vi "LV FPGA Serial Read Write v1_1.vi"(5 "Receive":refnum<k21>="ConnectorA/DIO10", 7 "baud rate (9600)":u32=31250, 9 "data bits (8)":i32=8 min=5 max=8 step=1, 11 "parity (0:none)":enum16{"None", "Odd", "Even", "Mark", "Space"}(ring), 12 "stop bits (10: 1 bit)":u16(ring)=10 items=["1.0"=10, "1.5"=15, "2.0"=20], 13 "Invert Polarity?":bool) -> ()   [LabVIEW 2014]
uses:
  <vilib>/rvi/Emulation/niFpgaGetClockAttributes.vi
  <vilib>/rvi/Emulation/niFpgaSctlEmulationGetInTimedLoop.vi
  <vilib>/rvi/Emulation/niFpgaEmulationReportErrorSimple.vi
  <vilib>/rvi/Emulation/niFpgaProcessEmulError.vi
  Controls/Stop.vi
  <vilib>/rvi/eio/common/nirviEmuTemplateMethod_errors.vi
  <vilib>/rvi/Emulation/niFpgaCriticalErrorInLSC.vi
  <vilib>/rvi/Emulation/niFpgaEmulationIsFPGAContextNoSignature.vi
  <vilib>/rvi/errors/niFpgaSetErrorForExecOnDevCompSimple.vi
  <vilib>/rvi/eio/common/nirviEmuReportErrorAndStop.vi
  <vilib>/rvi/DataTransferAndStorage/Container/Common/niFpgaContainerGetUniqueNameForEmu.vi
  <vilib>/rvi/FIFO/Fifo_Resource/nirvififoEmulationSetSize.vi
  <vilib>/rvi/FIFO/Fifo_Resource/nirviFifoEmulationQueueMgr.vi
  <instcachedir>/0/nirviFifoEmulationQueueMgr_E5CAEC123FF24DC58D834DCA3CDAA9B5.lvgen/nirviFifoEmulationQueueMgr_E5CAEC123FF24DC58D834DCA3CDAA9B5_000.vi
  <vilib>/rvi/FIFO/Fifo_Resource/nirvififoEmulationDetermineInputValidOut.vi
  <vilib>/rvi/FIFO/Fifo_Resource/nirvififoEmulationCreateLock.vi
  <vilib>/rvi/FIFO/Fifo_Resource/nirvififoEmulationObtainLock.vi
  <vilib>/rvi/FIFO/Fifo_Resource/nirvififoEmulationReleaseLock.vi
  <vilib>/rvi/occurrence/nirviWaitOnOccurrenceBase.vi
  <vilib>/rvi/errors/nirviReportUnexpectedCaseInternalError.vi
  <vilib>/rvi/errors/nirviReportUnexpectedCaseInternalError (U32).vi
  <vilib>/eio/EIONode/EIONode.xnode
  <vilib>/rvi/DataTransferAndStorage/Container/XNode/niFpgaContainer.xnode
  <vilib>/rvi/FIFO/Fifo_Resource/nirvififoEmulationWrite.vi
panel:
  out "Read: Transmission Error":bool
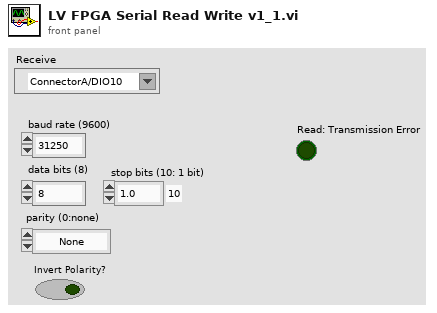
[diagram p1: front panel]
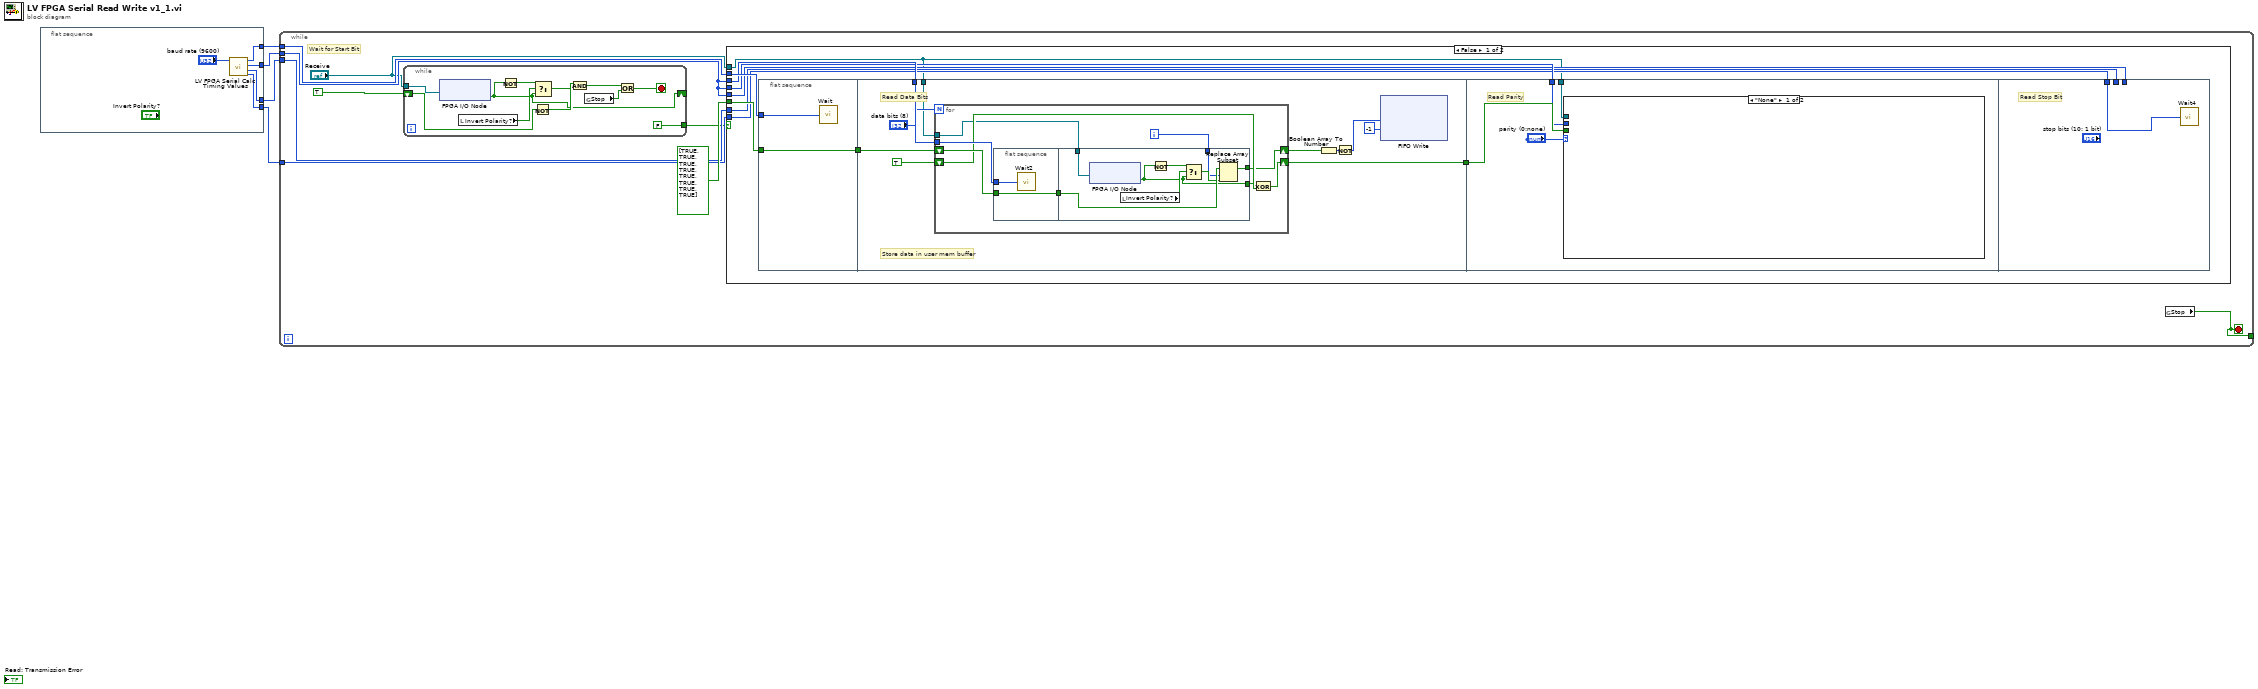
[diagram p0: block diagram]
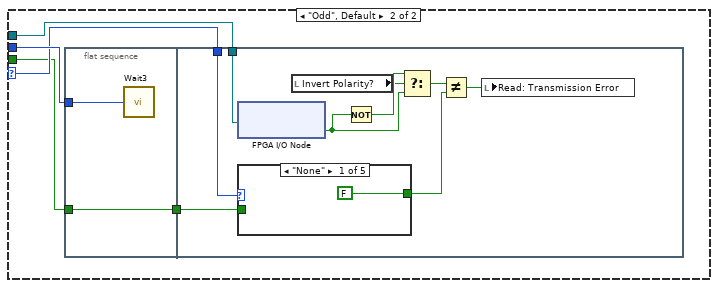
[diagram p2: hidden frame]
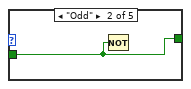
[diagram p3: hidden frame]
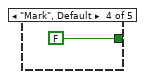
[diagram p5: hidden frame]
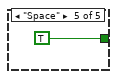
[diagram p6: hidden frame]
diagram:
  n1 = flat-sequence {
    tunnel: [w5] -> w3
    tunnel: [w8] -> w4
    tunnel: [w7] -> w2
    tunnel: [w6] -> w1
    frame #0 {
      n2 = call "LV FPGA Serial Calc Timing Values.vi"("baud rate (1000000)"="baud rate (9600)") -> ("Two Bit"=w6:u32, "One and Half Bit"=w7:u32, "One Bit"=w5:u32, "Half Bit"=w8:u32)  [unwired: 1 in, 2 out]
    }
  }
  n3 = while {
    tunnel: w1 -> [w17]
    tunnel: w2 -> [w16]
    tunnel: w3 -> [w15]
    tunnel: w4 -> [w14]
    tunnel: [w10] -> _
    stop <- w10 stop-if-true
    # "Wait for Start Bit"
    n4 = while {
      tunnel: [FALSE] -> w13
      shift-right: [w20] -> _
      shift-left: TRUE -> [w28]
      tunnel: "Receive" -> [w24]
      stop <- w25 stop-if-true
      n5 = xnode "FPGA I/O Node"("FPGA I/O In"=w24) -> ("I/O Item"=w20:bool)  [unwired: 1 out]
      n6 = local read "Invert Polarity?"() -> (w22:bool)
      n7 = Not(x=w20) -> (.not. x?=w23:bool)
      n8 = Not(x=w28) -> (.not. x?=w27:bool)
      n9 = Select(t=w23, s=w22, f=w20) -> (s? t:f=w21:bool)
      n10 = And(x=w27, y=w21) -> (x .and. y?=w26:bool)
      n11 = global read "Stop.vi" "Stop"() -> (w19:bool)
      n12 = Or(x=w26, y=w19) -> (x .or. y?=w25:bool)
    }
    n13 = case shown="False" w13 {
      tunnel: bool[] [TRUE, TRUE, TRUE, TRUE, TRUE, TRUE, TRUE, TRUE] -> [w38 _]
      tunnel: w14 -> [w37 _]
      tunnel: w15 -> [w36 _]
      tunnel: w15 -> [w35 _]
      tunnel: w15 -> [w34 _]
      tunnel: w16 -> [w33 _]
      tunnel: w17 -> [w32 _]
      tunnel: "Receive" -> [w30 _]
      frame False {
        n14 = flat-sequence {
          tunnel: [w41] -> w39
          tunnel: w38 -> [w41]
          tunnel: w37 -> [w40]
          tunnel: w39 -> [w51]
          tunnel: w36 -> [w50]
          tunnel: [w48] -> w31
          tunnel: w30 -> [w46]
          tunnel: w35 -> [w72]
          tunnel: w31 -> [w74]
          tunnel: w30 -> [w71]
          tunnel: w34 -> [_]
          tunnel: w33 -> [_]
          tunnel: w32 -> [w96]
          frame #0 {
            n15 = call "Wait"("Count(Ticks)"=w40) -> ()  [unwired: 1 out]
          }
          frame #1 {
            # "Store data in user mem buffer"
            # "Read Data Bits"
            n16 = for {
              N: "data bits (8)" -> [_]
              shift-right: [w54] -> w42
              shift-left: w51 -> [w60]
              tunnel: w50 -> [w58]
              shift-right: [w57] -> w48
              shift-left: TRUE -> [w56]
              tunnel: w46 -> [w53]
              i -> [w52]
              n17 = flat-sequence {
                tunnel: w60 -> [w62]
                tunnel: [w62] -> w59
                tunnel: w58 -> [w61]
                tunnel: w59 -> [w70]
                tunnel: [w69] -> w54
                tunnel: [w64] -> w55
                tunnel: w53 -> [w68]
                tunnel: w52 -> [w63]
                frame #0 {
                  n18 = call "Wait2"("Count(Ticks)"=w61) -> ()  [unwired: 1 out]
                }
                frame #1 {
                  n19 = xnode "FPGA I/O Node"("FPGA I/O In"=w68) -> ("I/O Item"=w64:bool)  [unwired: 1 out]
                  n20 = local read "Invert Polarity?"() -> (w67:bool)
                  n21 = Not(x=w64) -> (.not. x?=w66:bool)
                  n22 = Select(t=w66, s=w67, f=w64) -> (s? t:f=w65:bool)
                  n23 = Replace Array Subset(array=w70, new element=w65, index=w63) -> (w69:bool[])
                }
              }
              n24 = Exclusive Or(1:w56, 2:w55) -> (0:w57:bool)
            }
            n25 = Boolean Array To Number(Boolean array=w42) -> (number=w44:u8)
            n26 = Not(x=w44) -> (.not. x?=w43:u8)
            n27 = xnode ("FIFO Write")("Element"=w43, "Timeout"=-1) -> ()  [unwired: 1 in, 2 out]
          }
          frame #2 {
            # "Read Parity"
            n28 = case shown="\"None\"" "parity (0:none)" {
              selector: "parity (0:none)" -> [_ w78]
              tunnel: w74 -> [_ w76]
              tunnel: w72 -> [_ w79]
              tunnel: w71 -> [_ w75]
              frame "None" {
              }
              frame "Odd", Default {
                n29 = flat-sequence {
                  tunnel: w79 -> [w81]
                  tunnel: [w80] -> w77
                  tunnel: w76 -> [w80]
                  tunnel: w78 -> [w90]
                  tunnel: w77 -> [w88]
                  tunnel: w75 -> [w86]
                  frame #0 {
                    n30 = call "Wait3"("Count(Ticks)"=w81) -> ()  [unwired: 1 out]
                  }
                  frame #1 {
                    n31 = xnode "FPGA I/O Node"("FPGA I/O In"=w86) -> ("I/O Item"=w83:bool)  [unwired: 1 out]
                    n32 = case shown="\"None\"" w90 {
                      tunnel: w88 -> [_ w92 w93 _ _]
                      tunnel: [FALSE ("y") w92 w93 FALSE ("y") TRUE ("y")] -> w89
                      frame "None" {
                      }
                      frame "Odd" {
                        n33 = Not(x=w92) -> ()  [unwired: 1 out]
                      }
                      frame "Even" {
                      }
                      frame "Mark", Default {
                      }
                      frame "Space" {
                      }
                    }
                    n34 = local read "Invert Polarity?"() -> (w84:bool)
                    n35 = Not(x=w83) -> (.not. x?=w85:bool)
                    n36 = Select(t=w85, s=w84, f=w83) -> (s? t:f=w82:bool)
                    n37 = Not Equal?(x=w82, y=w89) -> (x != y?=w87:bool)
                    n38 = local write "Read: Transmission Error"(w87) -> ()
                  }
                }
              }
            }
          }
          frame #3 {
            # "Read Stop Bit"
            n39 = call "Wait4"("Count(Ticks)"=w96) -> ()  [unwired: 1 out]
          }
        }
      }
      frame True {
      }
    }
    n40 = global read "Stop.vi" "Stop"() -> (w10:bool)
  }
